vi "Convert from 2s Complement.vi"(10 "number of bits":i32, 11 "data":u32[][](array[numeric])) -> (3 "data out":i32[][](array[numeric]))   [LabVIEW 2021]
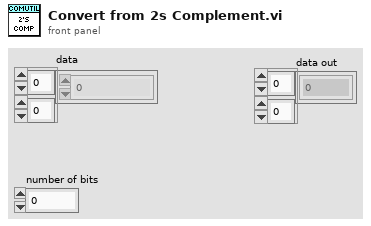
[diagram p1: front panel]
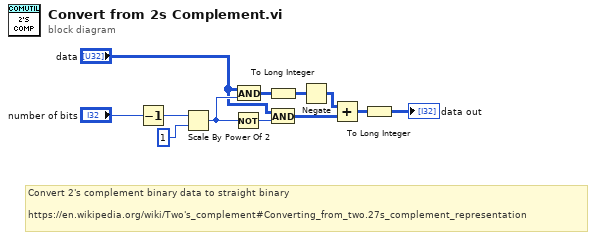
[diagram p0: block diagram]
diagram:
  # "Convert 2's complement binary data to straight binary\n\nhttps://en.wikipedia.org/wiki/Two's_complement#Converting_from_two.27s_complement_representation"
  n1 = Decrement(x="number of bits") -> (x-1=w6:i32)
  n2 = Scale By Power Of 2(n=w6, x=u32 1) -> (x*2^n=w4:u32)
  n3 = Not(x=w4) -> (.not. x?=w11:u32)
  n4 = And(x="data", y=w4) -> (x .and. y?=w8:u32[][])
  n5 = To Long Integer(number=w8) -> (32bit integer=w7:i32[][])
  n6 = And(x="data", y=w11) -> (x .and. y?=w10:u32[][])
  n7 = Negate(x=w7) -> (-x=w12:i32[][])
  n8 = Add(x=w12, y=w10) -> (x+y=w9:u32[][])
  n9 = To Long Integer(number=w9) -> (32bit integer=→"data out":i32[][])
